vi "Generic command handler.vi"(8 "error in (no error)":errorcluster, 10 "Message in":refnum<class "GenericMessage.lvclass">, 11 "StageSPIM in":refnum<class "StageSPIM.lvclass">) -> (0 "error out":errorcluster, 2 "value":string, 3 "StageSPIM out":refnum<class "StageSPIM.lvclass">)   [LabVIEW 2012, in "StageSPIM.lvclass"]
doc: "The generic_command_handler processes the command 'generic'. Commands which are not part of the predefined list of commands fall under the 'generic' command for special activity."
uses:
  StageSPIM.lvclass
  <vilib>/Distrio/Murmex/GenericMessage/GenericMessage.lvclass
  <vilib>/Distrio/Murmex/Murmex/Murmex.lvclass
  StageSPIM.lvclass/StageSPIM.ctl
  <vilib>/Distrio/Murmex/ProceedMessage/ProceedMessage.lvclass
  <vilib>/Distrio/Murmex/Message/Message.lvclass
panel:
  # "This method is called when the GENERIC\ntrigger is sent. \n\nOverride this method when your component needs to\nrespond to this trigger. \n\nCall parent for proper implementation"
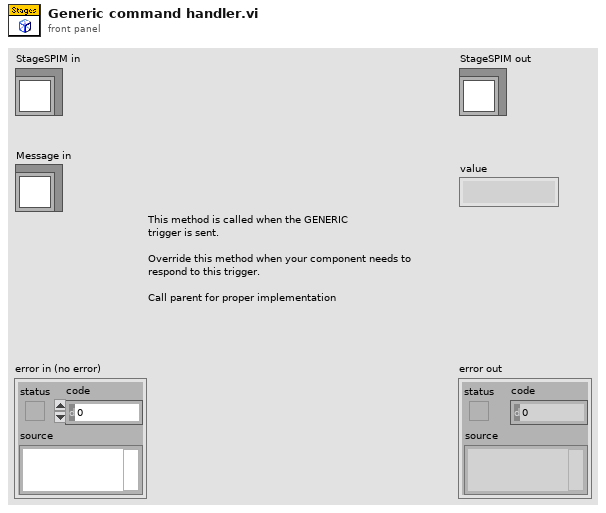
[diagram p1: front panel]
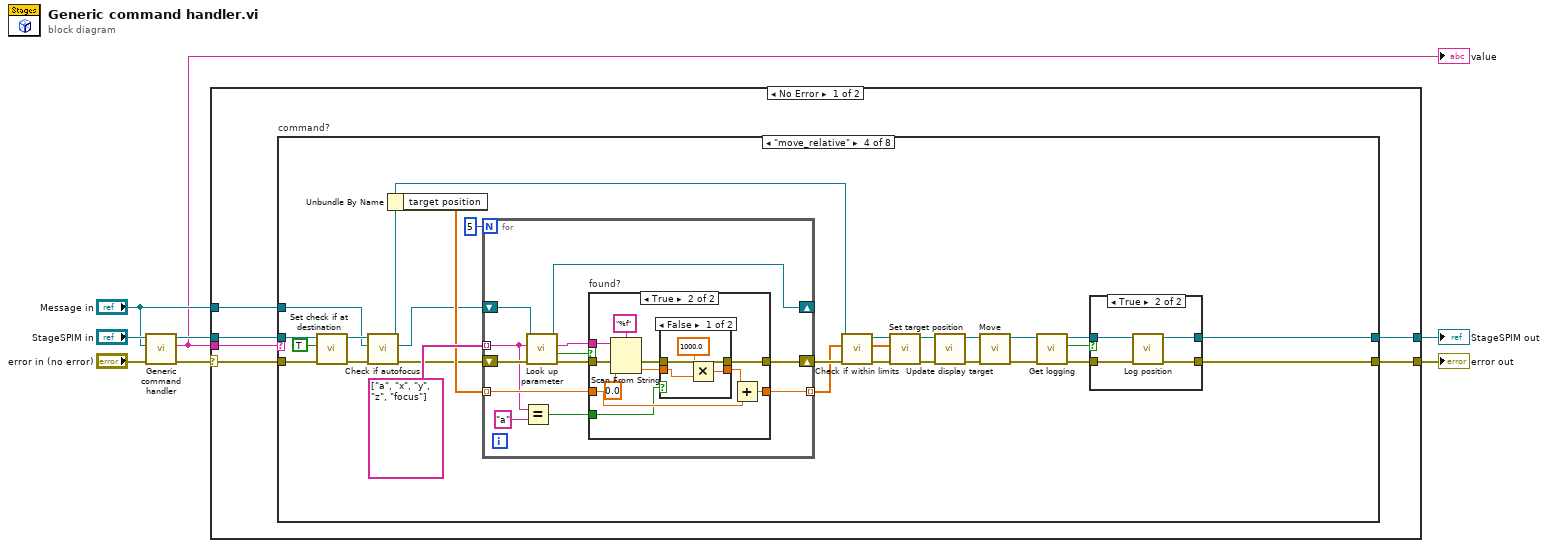
[diagram p0: block diagram]
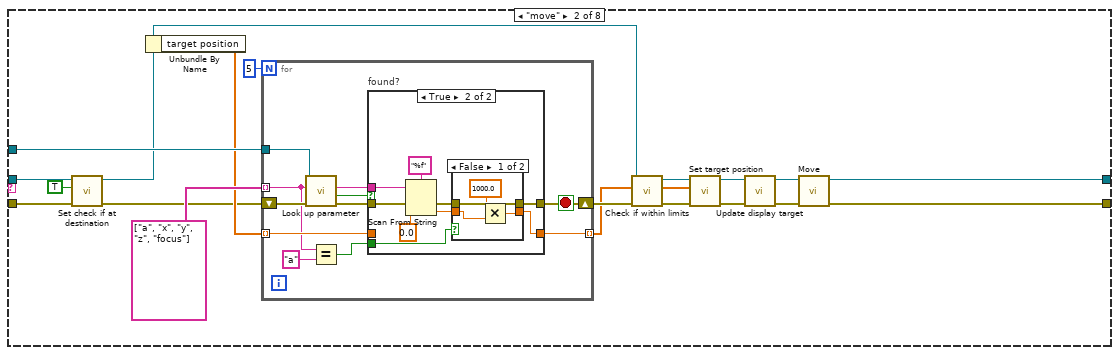
[diagram p3: hidden frame]
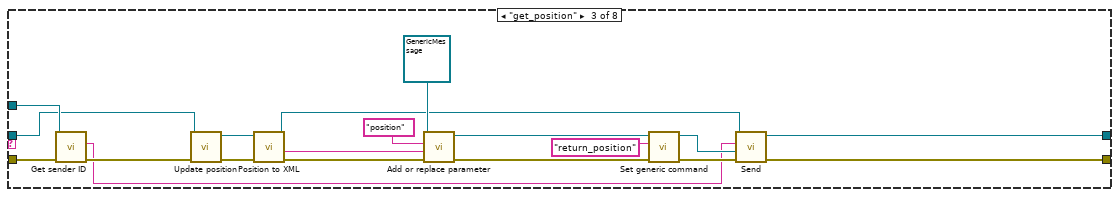
[diagram p6: hidden frame]
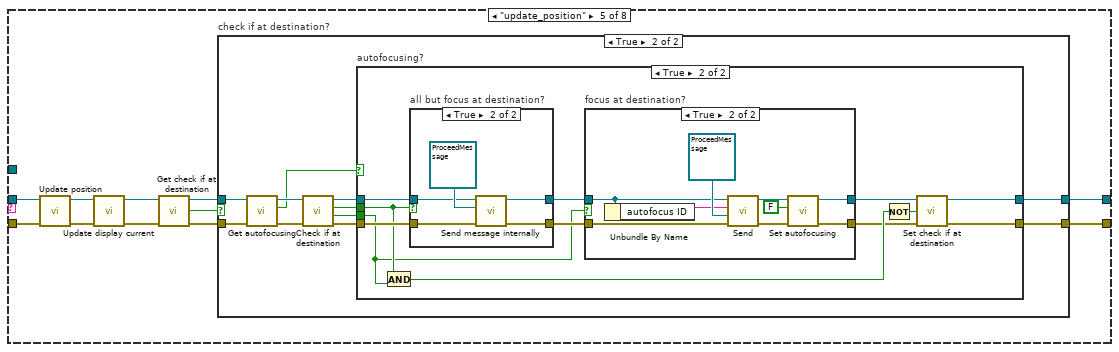
[diagram p10: hidden frame]
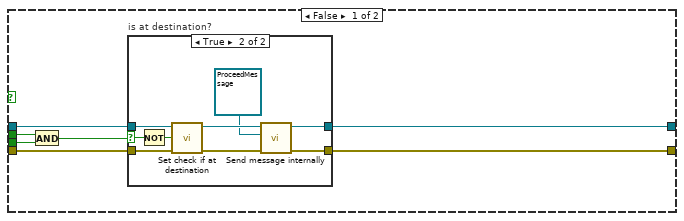
[diagram p12: hidden frame]
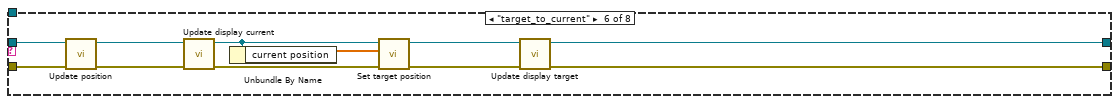
[diagram p16: hidden frame]
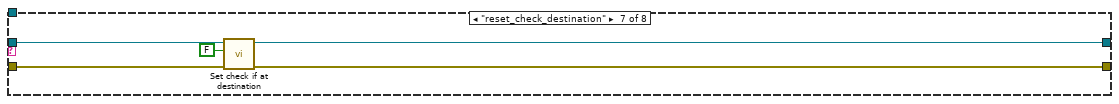
[diagram p17: hidden frame]
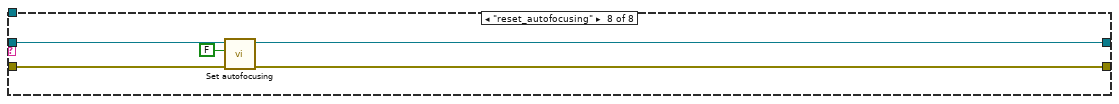
[diagram p18: hidden frame]
diagram:
  n1 = call-parent "Generic command handler.vi"("error in (no error)"="error in (no error)", "Message in"="Message in", "Murmex in"="StageSPIM in") -> ("error out"=w6:errorcluster, "value"=w3:string, "Murmex out"=w5:refnum<class "StageSPIM.lvclass">)  [unwired: 6 in]
  "value" <- w3
  n2 = case shown="No Error" w6 {
    selector: w6 -> [w13 w242]
    tunnel: w3 -> [w14 _]
    tunnel: w5 -> [w12 w243]
    tunnel: "Message in" -> [w11 _]
    tunnel: [w10 w242] -> w2
    tunnel: [w9 w243] -> w1
    frame No Error {
      n3 = case "command?" shown="\"move_relative\"" w14 {
        tunnel: w13 -> [w15 w26 w83 w103 w159 w229 w236 w241]
        tunnel: w12 -> [w16 w28 w69 w104 w158 w228 w235 w240]
        tunnel: w11 -> [_ w33 w82 w92 _ _ _ _]
        tunnel: [w15 w18 w65 w85 w153 w223 w232 w238] -> w10
        tunnel: [w16 w19 w66 w86 w154 w221 w233 w239] -> w9
        frame Default {
        }
        frame "move" {
          n4 = call-dynamic "Set check if at destination.vi"("error in (no error)"=w26, "check if at destination"=TRUE, "StageSPIM in"=w28) -> ("error out"=w25:errorcluster, "StageSPIM out"=w27:refnum<class "StageSPIM.lvclass">)  [unwired: 7 in]
          n5 = Unbundle By Name(w27) -> ("target position"=w30:dbl[])
          n6 = for {
            N: 5 -> [_]
            shift-right: [w40] -> w34
            shift-left: w25 -> [w47]
            tunnel: string[] ["a", "x", "y", "z", "focus"] -> [w38] mode=indexing
            tunnel: w30 -> [w42] mode=indexing
            tunnel: [w41] -> w29 mode=indexing
            tunnel: w33 -> [w43]
            stop <- w40 stop-if-true
            n7 = call <vilib>:"Look up parameter.vi"("error in (no error)"=w47, "name"=w38, "Message in"=w43) -> ("error out"=w46:errorcluster, "found?"=w45:bool, "key"=w44:string)  [unwired: 5 in, 1 out]
            n8 = Equal?(x=w38, y="a") -> (x = y?=w37:bool)
            n9 = case "found?" shown="True" w45 {
              tunnel: w46 -> [w49 w58]
              tunnel: [w49 w53] -> w40
              tunnel: w44 -> [_ w56]
              tunnel: [w48 w51] -> w41
              tunnel: w42 -> [w48 _]
              tunnel: w37 -> [_ w50]
              frame False {
              }
              frame True {
                n10 = Scan From String(format string="%f", input string=w56, error in=w58, default 1=0.0 ("default value 1")) -> (error out=w54:errorcluster, output 1=w52:dbl)  [unwired: 1 in, 2 out]
                n11 = case shown="False" w50 {
                  tunnel: [w62 w64] -> w53
                  tunnel: w54 -> [w62 w64]
                  tunnel: [w61 w63] -> w51
                  tunnel: w52 -> [w60 w63]
                  frame False {
                    n12 = Multiply(x=1000.0, y=w60) -> (x*y=w61:dbl)
                  }
                  frame True {
                  }
                }
              }
            }
          }
          n13 = call-dynamic "Check if within limits.vi"("error in (no error)"=w34, "Position array in"=w29, "StageSPIM in"=w27) -> ("error out"=w35:errorcluster, "Approved postion array"=w17:dbl[], "StageSPIM out"=w36:refnum<class "StageSPIM.lvclass">)  [unwired: 4 in, 2 out]
          n14 = call-dynamic "Set target position.vi"("error in (no error)"=w35, "target position"=w17, "StageSPIM in"=w36) -> ("error out"=w23:errorcluster, "StageSPIM out"=w21:refnum<class "StageSPIM.lvclass">)  [unwired: 7 in]
          n15 = call-dynamic "Update display target.vi"("error in (no error)"=w23, "StageSPIM in"=w21) -> ("error out"=w22:errorcluster, "StageSPIM out"=w20:refnum<class "StageSPIM.lvclass">)  [unwired: 8 in]
          n16 = call-dynamic "Move.vi"("error in (no error)"=w22, "StageSPIM in"=w20) -> ("error out"=w18:errorcluster, "StageSPIM out"=w19:refnum<class "StageSPIM.lvclass">)  [unwired: 8 in]
        }
        frame "get_position" {
          n17 = call <vilib>:"Get sender ID.vi"("error in (no error)"=w83, "Message in"=w82) -> ("error out"=w81:errorcluster, "sender"=w77:string)  [unwired: 7 in, 1 out]
          n18 = call-dynamic "Update position.vi"("error in (no error)"=w81, "StageSPIM in"=w69) -> ("error out"=w71:errorcluster, "StageSPIM out"=w68:refnum<class "StageSPIM.lvclass">)  [unwired: 8 in]
          n19 = call-dynamic "Position to XML.vi"("error in (no error)"=w71, "StageSPIM in"=w68) -> ("error out"=w70:errorcluster, "XML string"=w67:string, "StageSPIM out"=w72:refnum<class "StageSPIM.lvclass">)  [unwired: 7 in]
          n20 = call <vilib>:"Add or replace parameter.vi"("error in (no error)"=w70, "value"=w67, "name"="position", "Message in"=refnum<class "GenericMessage.lvclass"> refnum ("Distrio Murmex 1.1:GenericMessage")) -> ("error out"=w75:errorcluster, "Message out"=w74:refnum<class "GenericMessage.lvclass">)  [unwired: 6 in]
          n21 = call <vilib>:"Set generic command.vi"("error in (no error)"=w75, "generic command"="return_position", "GenericMessage in"=w74) -> ("error out"=w79:errorcluster, "GenericMessage out"=w78:refnum<class "GenericMessage.lvclass">)  [unwired: 7 in]
          n22 = call <vilib>:"Send.vi"("error in (no error)"=w79, "Message"=w78, "recipient"=w77, "Murmex in"=w72) -> ("error out"=w65:errorcluster, "Murmex out"=w66:refnum<class "StageSPIM.lvclass">)  [unwired: 6 in]
        }
        frame "move_relative" {
          n23 = call-dynamic "Set check if at destination.vi"("error in (no error)"=w103, "check if at destination"=TRUE, "StageSPIM in"=w104) -> ("error out"=w96:errorcluster, "StageSPIM out"=w94:refnum<class "StageSPIM.lvclass">)  [unwired: 7 in]
          n24 = call-dynamic "Check if autofocus.vi"("error in (no error)"=w96, "Message in"=w92, "StageSPIM in"=w94) -> ("error out"=w95:errorcluster, "Message out"=w91:refnum<class "GenericMessage.lvclass">, "StageSPIM out"=w93:refnum<class "StageSPIM.lvclass">)  [unwired: 6 in]
          n25 = Unbundle By Name(w93) -> ("target position"=w106:dbl[])
          n26 = for {
            N: 5 -> [_]
            shift-right: [w126] -> w109
            shift-left: w95 -> [w129]
            tunnel: string[] ["a", "x", "y", "z", "focus"] -> [w120] mode=indexing
            shift-right: [w123] -> _
            shift-left: w91 -> [w124]
            tunnel: w106 -> [w122] mode=indexing
            tunnel: [w121] -> w105 mode=indexing
            n27 = Equal?(x=w120, y="a") -> (x = y?=w118:bool)
            n28 = call <vilib>:"Look up parameter.vi"("error in (no error)"=w129, "name"=w120, "Message in"=w124) -> ("error out"=w128:errorcluster, "found?"=w127:bool, "key"=w125:string, "Message out"=w123:refnum<class "GenericMessage.lvclass">)  [unwired: 5 in]
            n29 = case "found?" shown="True" w127 {
              tunnel: w128 -> [w131 w142]
              tunnel: [w131 w135] -> w126
              tunnel: w125 -> [_ w140]
              tunnel: [w130 w138] -> w121
              tunnel: w122 -> [w130 w137]
              tunnel: w118 -> [_ w136]
              frame False {
              }
              frame True {
                n30 = Scan From String(format string="%f", input string=w140, error in=w142, default 1=0.0 ("default value 1")) -> (error out=w134:errorcluster, output 1=w132:dbl)  [unwired: 1 in, 2 out]
                n31 = case shown="False" w136 {
                  tunnel: [w146 w148] -> w135
                  tunnel: w134 -> [w146 w148]
                  tunnel: [w145 w147] -> w133
                  tunnel: w132 -> [w144 w147]
                  frame False {
                    n32 = Multiply(x=1000.0, y=w144) -> (x*y=w145:dbl)
                  }
                  frame True {
                  }
                }
                n33 = Add(x=w133, y=w137) -> (x+y=w138:dbl)
              }
            }
          }
          n34 = call-dynamic "Check if within limits.vi"("error in (no error)"=w109, "Position array in"=w105, "StageSPIM in"=w93) -> ("error out"=w110:errorcluster, "Approved postion array"=w84:dbl[], "StageSPIM out"=w111:refnum<class "StageSPIM.lvclass">)  [unwired: 4 in, 2 out]
          n35 = call-dynamic "Set target position.vi"("error in (no error)"=w110, "target position"=w84, "StageSPIM in"=w111) -> ("error out"=w100:errorcluster, "StageSPIM out"=w97:refnum<class "StageSPIM.lvclass">)  [unwired: 7 in]
          n36 = call-dynamic "Update display target.vi"("error in (no error)"=w100, "StageSPIM in"=w97) -> ("error out"=w99:errorcluster, "StageSPIM out"=w98:refnum<class "StageSPIM.lvclass">)  [unwired: 8 in]
          n37 = call-dynamic "Move.vi"("error in (no error)"=w99, "StageSPIM in"=w98) -> ("error out"=w101:errorcluster, "StageSPIM out"=w87:refnum<class "StageSPIM.lvclass">)  [unwired: 8 in]
          n38 = call-dynamic "Get logging.vi"("error in (no error)"=w101, "StageSPIM in"=w87) -> ("error out"=w89:errorcluster, "logging?"=w90:bool, "StageSPIM out"=w88:refnum<class "StageSPIM.lvclass">)  [unwired: 7 in]
          n39 = case shown="True" w90 {
            tunnel: w89 -> [w113 w117]
            tunnel: w88 -> [w112 w116]
            tunnel: [w113 w114] -> w85
            tunnel: [w112 w115] -> w86
            frame False {
            }
            frame True {
              n40 = call-dynamic "Log position.vi"("error in (no error)"=w117, "StageSPIM in"=w116) -> ("error out"=w114:errorcluster, "StageSPIM out"=w115:refnum<class "StageSPIM.lvclass">)  [unwired: 8 in]
            }
          }
        }
        frame "update_position" {
          n41 = call-dynamic "Update position.vi"("error in (no error)"=w159, "StageSPIM in"=w158) -> ("error out"=w152:errorcluster, "StageSPIM out"=w150:refnum<class "StageSPIM.lvclass">)  [unwired: 8 in]
          n42 = call-dynamic "Update display current.vi"("error in (no error)"=w152, "StageSPIM in"=w150) -> ("error out"=w151:errorcluster, "StageSPIM out"=w149:refnum<class "StageSPIM.lvclass">)  [unwired: 8 in]
          n43 = call-dynamic "Get check if at destination.vi"("error in (no error)"=w151, "StageSPIM in"=w149) -> ("error out"=w156:errorcluster, "check if at destination"=w157:bool, "StageSPIM out"=w155:refnum<class "StageSPIM.lvclass">)  [unwired: 7 in]
          n44 = case "check if at destination?" shown="True" w157 {
            tunnel: w156 -> [w161 w167]
            tunnel: w155 -> [w160 w165]
            tunnel: [w160 w169] -> w154
            tunnel: [w161 w168] -> w153
            frame False {
            }
            frame True {
              n45 = call-dynamic "Get autofocusing.vi"("error in (no error)"=w167, "StageSPIM in"=w165) -> ("error out"=w166:errorcluster, "autofocusing?"=w163:bool, "StageSPIM out"=w164:refnum<class "StageSPIM.lvclass">)  [unwired: 7 in]
              n46 = call-dynamic "Check if at destination.vi"("error in (no error)"=w166, "StageSPIM in"=w164) -> ("error out"=w171:errorcluster, "focus at destination?"=w162:bool, "at destination? (all but focus)"=w172:bool, "StageSPIM out"=w170:refnum<class "StageSPIM.lvclass">)  [unwired: 6 in]
              n47 = case "autofocusing?" shown="True" w163 {
                tunnel: w172 -> [w175 w198]
                tunnel: w171 -> [w179 w202]
                tunnel: w170 -> [w178 w201]
                tunnel: [w177 w191] -> w169
                tunnel: [w176 w193] -> w168
                tunnel: w162 -> [w174 w197]
                frame False {
                  n48 = And(x=w175, y=w174) -> (x .and. y?=w173:bool)
                  n49 = case "is at destination?" shown="True" w173 {
                    selector: w173 -> [_ w189]
                    tunnel: w179 -> [w181 w190]
                    tunnel: w178 -> [w180 w187]
                    tunnel: [w181 w183] -> w176
                    tunnel: [w180 w182] -> w177
                    frame False {
                    }
                    frame True {
                      n50 = Not(x=w189) -> (.not. x?=w188:bool)
                      n51 = call-dynamic "Set check if at destination.vi"("error in (no error)"=w190, "check if at destination"=w188, "StageSPIM in"=w187) -> ("error out"=w186:errorcluster, "StageSPIM out"=w185:refnum<class "StageSPIM.lvclass">)  [unwired: 7 in]
                      n52 = call <vilib>:"Send message internally.vi"("error in (no error)"=w186, "Message"=refnum<class "ProceedMessage.lvclass"> refnum ("Distrio Murmex 1.1:ProceedMessage"), "Murmex in"=w185) -> ("error out"=w183:errorcluster, "Murmex out"=w182:refnum<class "StageSPIM.lvclass">)  [unwired: 7 in]
                    }
                  }
                }
                frame True {
                  n53 = And(x=w198, y=w197) -> (x .and. y?=w195:bool)
                  n54 = case "all but focus at destination?" shown="True" w198 {
                    tunnel: w202 -> [w215 w216]
                    tunnel: w201 -> [w214 w217]
                    tunnel: [w215 w219] -> w199
                    tunnel: [w214 w218] -> w200
                    frame False {
                    }
                    frame True {
                      n55 = call <vilib>:"Send message internally.vi"("error in (no error)"=w216, "Message"=refnum<class "ProceedMessage.lvclass"> refnum ("Distrio Murmex 1.1:ProceedMessage"), "Murmex in"=w217) -> ("error out"=w219:errorcluster, "Murmex out"=w218:refnum<class "StageSPIM.lvclass">)  [unwired: 7 in]
                    }
                  }
                  n56 = case "focus at destination?" shown="True" w197 {
                    tunnel: w199 -> [w204 w213]
                    tunnel: w200 -> [w203 w210]
                    tunnel: [w204 w208] -> w194
                    tunnel: [w203 w206] -> w192
                    frame False {
                    }
                    frame True {
                      n57 = Unbundle By Name(w210) -> ("autofocus ID"=w209:string)
                      n58 = call <vilib>:"Send.vi"("error in (no error)"=w213, "Message"=refnum<class "ProceedMessage.lvclass"> refnum ("Distrio Murmex 1.1:ProceedMessage"), "recipient"=w209, "Murmex in"=w210) -> ("error out"=w212:errorcluster, "Murmex out"=w207:refnum<class "StageSPIM.lvclass">)  [unwired: 6 in]
                      n59 = call-dynamic "Set autofocusing.vi"("error in (no error)"=w212, "autofocusing?"=FALSE, "StageSPIM in"=w207) -> ("error out"=w208:errorcluster, "StageSPIM out"=w206:refnum<class "StageSPIM.lvclass">)  [unwired: 7 in]
                    }
                  }
                  n60 = Not(x=w195) -> (.not. x?=w196:bool)
                  n61 = call-dynamic "Set check if at destination.vi"("error in (no error)"=w194, "check if at destination"=w196, "StageSPIM in"=w192) -> ("error out"=w193:errorcluster, "StageSPIM out"=w191:refnum<class "StageSPIM.lvclass">)  [unwired: 7 in]
                }
              }
            }
          }
        }
        frame "target_to_current" {
          n62 = call-dynamic "Update position.vi"("error in (no error)"=w229, "StageSPIM in"=w228) -> ("error out"=w231:errorcluster, "StageSPIM out"=w230:refnum<class "StageSPIM.lvclass">)  [unwired: 8 in]
          n63 = call-dynamic "Update display current.vi"("error in (no error)"=w231, "StageSPIM in"=w230) -> ("error out"=w226:errorcluster, "StageSPIM out"=w227:refnum<class "StageSPIM.lvclass">)  [unwired: 8 in]
          n64 = Unbundle By Name(w227) -> ("current position"=w225:dbl[])
          n65 = call-dynamic "Set target position.vi"("error in (no error)"=w226, "target position"=w225, "StageSPIM in"=w227) -> ("error out"=w224:errorcluster, "StageSPIM out"=w222:refnum<class "StageSPIM.lvclass">)  [unwired: 7 in]
          n66 = call-dynamic "Update display target.vi"("error in (no error)"=w224, "StageSPIM in"=w222) -> ("error out"=w223:errorcluster, "StageSPIM out"=w221:refnum<class "StageSPIM.lvclass">)  [unwired: 8 in]
        }
        frame "reset_check_destination" {
          n67 = call-dynamic "Set check if at destination.vi"("error in (no error)"=w236, "check if at destination"=FALSE, "StageSPIM in"=w235) -> ("error out"=w232:errorcluster, "StageSPIM out"=w233:refnum<class "StageSPIM.lvclass">)  [unwired: 7 in]
        }
        frame "reset_autofocusing" {
          n68 = call-dynamic "Set autofocusing.vi"("error in (no error)"=w241, "autofocusing?"=FALSE ("check if at destination"), "StageSPIM in"=w240) -> ("error out"=w238:errorcluster, "StageSPIM out"=w239:refnum<class "StageSPIM.lvclass">)  [unwired: 7 in]
        }
      }
    }
    frame Error {
    }
  }
  "error out" <- w2
  "StageSPIM out" <- w1
